vi "Servo_init.vi"() -> (0 "error out":errorcluster)   [LabVIEW 2009, in "Servo.lvlib"]
uses:
  Servo.lvlib
  <vilib>/Utility/config.llb/Read Key (Double).vi
  <vilib>/Utility/config.llb/NI_LVConfig.lvlib
panel:
  out "Array":T1(array[cluster])
  in  "configuration file path":path
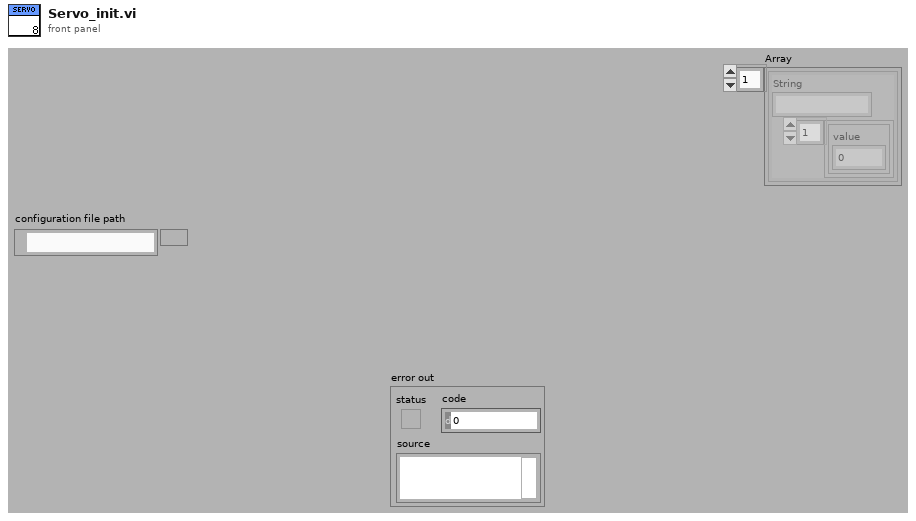
[diagram p1: front panel]
types:
  T1 = cluster{"String":string, cluster{"value":dbl}[]}[]
  T2 = typedef "NI_LVConfig.lvlib/Config Data RefNum.ctl" = refnum<k1>
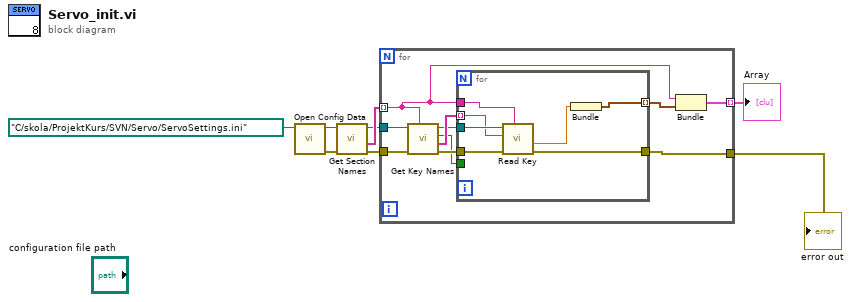
[diagram p0: block diagram]
diagram:
  n1 = call <vilib>:"Open Config Data.vi"("configuration file path"=path "C:/skola/ProjektKurs/SVN/Servo/ServoSettings.ini") -> ("error out"=w7:errorcluster, "refnum"=w8:T2)  [unwired: 8 in, 1 out]
  n2 = call <vilib>:"Get Section Names.vi"("error in (no error)"=w7, "refnum"=w8) -> ("error out"=w3:errorcluster, "section names"=w5:string[], "refnum out"=w4:T2)  [unwired: 7 in]
  n3 = for {
    tunnel: w5 -> [w11] mode=indexing
    tunnel: w4 -> [w14]
    tunnel: w3 -> [w13]
    tunnel: [w12] -> w2
    tunnel: [w10] -> w1 mode=indexing
    n4 = call <vilib>:"Get Key Names.vi"("section"=w11, "error in (no error)"=w13, "refnum"=w14) -> ("error out"=w17:errorcluster, "key names"=w18:string[], "section exists?"=w15:bool, "refnum out"=w16:T2)  [unwired: 5 in]
    n5 = for {
      tunnel: w18 -> [w22] mode=indexing
      tunnel: w17 -> [w25]
      tunnel: w16 -> [w24]
      tunnel: [w23] -> w12
      tunnel: w15 -> [_]
      tunnel: w11 -> [w21]
      tunnel: [w19] -> w9 mode=indexing
      n6 = call-poly <vilib>:"Read Key.vi"("section"=w21, "error in (no error)"=w25, "key"=w22, "refnum"=w24) -> ("error out"=w23:errorcluster, "value"=w20:dbl)  [unwired: 4 in, 2 out]
      n7 = Bundle("value"=w20) -> (w19:cluster{"value":dbl})  [unwired: 1 in]
    }
    n8 = Bundle("String"=w11, w9) -> (w10:cluster{"String":string, cluster{"value":dbl}[]})  [unwired: 1 in]
  }
  "error out" <- w2
  "Array" <- w1
